vi "Untitled 6.vi"(7 "error in (no error)":errorcluster) -> (0 "error out":errorcluster, 3 "CT-Stop-Cmd.lvclass":refnum<class "CT-Stop-Cmd.lvclass">)   [LabVIEW 2013, in "CT-Stop-Cmd.lvclass"]
uses:
  CT-Stop-Cmd.lvclass
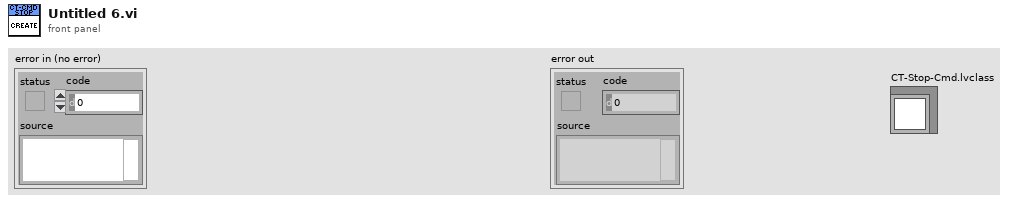
[diagram p1: front panel]
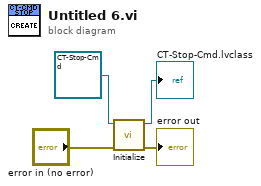
[diagram p0: block diagram]
diagram:
  n1 = call-dynamic "Initialize.vi"("error in (no error)"="error in (no error)", "CT-Stop-Cmd in"=refnum<class "CT-Stop-Cmd.lvclass"> refnum ("CT-Stop-Cmd.lvclass")) -> ("error out"=→"error out":errorcluster, "CT-Stop-Cmd out"=→"CT-Stop-Cmd.lvclass":refnum<class "CT-Stop-Cmd.lvclass">)  [unwired: 8 in]
